vi "Sort single measurements.vi"(1 "Table In":T1[](array[typedef]) {"Carrier_2 Q (l/min)" format="%#.2f"; "Row Duration (mins)" format="%#.1f"; "Row No" min=0; "Trace Gas Concentration (%)" min=0.0 format="%#_4f"; "Carrier_1 Q (l/min)" format="%#.2f"; "Tunnel Speed" format="%#.2f"; "Start X" format="%#.2f"; "Start Y" format="%#.2f"; "Start Z" format="%#.2f"; "End X" format="%#.2f"; "End Y" format="%#.2f"; "End Z" format="%#.2f"; "Averaging time (min)" min=0.0 format="%#.2f"}) -> (0 "Table Out":T1[](array[typedef]) {"Carrier_2 Q (l/min)" format="%#.2f"; "Row Duration (mins)" format="%#.1f"; "Row No" min=0; "Trace Gas Concentration (%)" min=0.0 format="%#_4f"; "Carrier_1 Q (l/min)" format="%#.2f"; "Tunnel Speed" format="%#.2f"; "Start X" format="%#.2f"; "Start Y" format="%#.2f"; "Start Z" format="%#.2f"; "End X" format="%#.2f"; "End Y" format="%#.2f"; "End Z" format="%#.2f"; "Averaging time (min)" min=0.0 format="%#.2f"})   [LabVIEW 2014]
uses:
  Anemometry Sub Vis/Gen Trav/Traverse_cluster.ctl
  Anemometry Sub Vis/Gen Trav/Spacing.ctl
  Anemometry Sub Vis/Controls/Multi_run_mode.ctl
panel:
  out "Stop":i32[](array[numeric])
  out "Start":i32[](array[numeric])
  # "X           Y            Z"
  # "Start"
  # "End"
  # "X           Y            Z"
  # "Start"
  # "End"
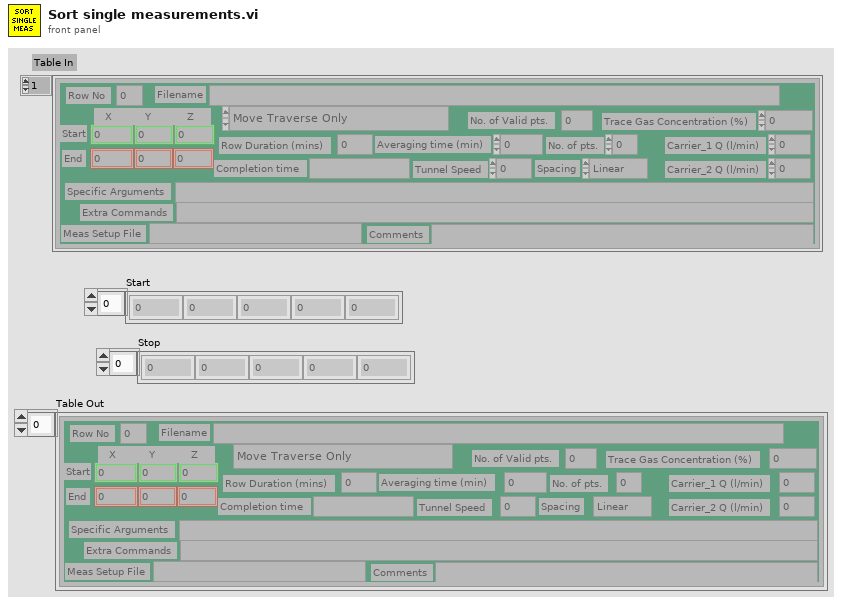
[diagram p1: front panel]
types:
  T1 = typedef "Traverse_cluster.ctl" = cluster{"Start X":sgl, "Start Y":sgl, "Start Z":sgl, "End X":sgl, "End Y":sgl, "End Z":sgl, "No. of pts.":i32, "Spacing":T2, "Filename":path, "Tunnel Speed":dbl, "Averaging time (min)":dbl, "Extra Commands":string, "Carrier_1 Q (l/min)":dbl, "Carrier_2 Q (l/min)":dbl, "Trace Gas Concentration (%)":dbl, "Specific Arguments":string, "Comments":string, "Row No":i32, "Row Type Selector":T3, "Completion time":string, "Row Duration (mins)":dbl, "No. of Valid pts.":i32, "Meas Setup File":string}
  T2 = typedef "Spacing.ctl" = enum16{"Linear", "Log", "Gauss", "Specified", "N/A"}
  T3 = typedef "Multi_run_mode.ctl" = enum16{"Move Traverse Only", "Set Tunnel Speed Only", "Set Source Only", "Set Measurement Conditions", "Single Measurement", "Vertical Profile", "Lateral Profile", "Longitudinal Profile", "Explore Volume", "Multi-Axis Profile", "Auto Calibrate", "Meas Fast FID Bkgnd", "Check Beam Power", "Scanning Valve Measurement", "Run VI Named:", "Set ADAM Ch", "Wait (minutes)", "Send Message", "Synchronize With:", "Fall Back to this Row", "Turn Off Row Repeating", "Blank Row", "Traverse 3D Volume"}
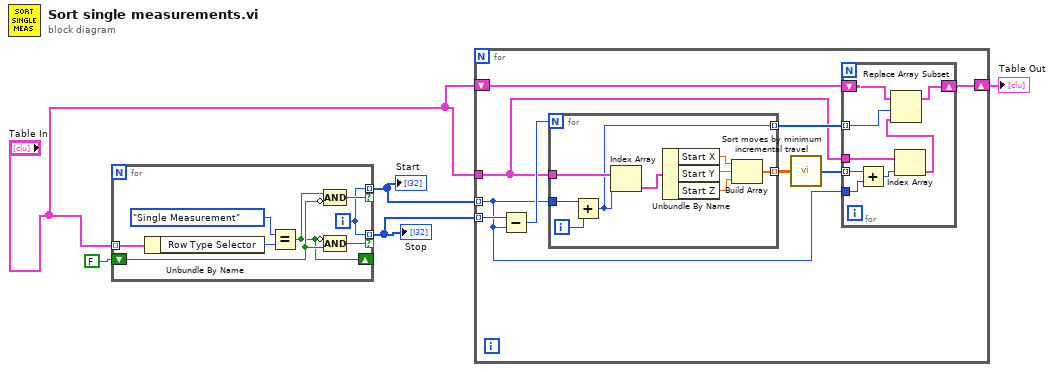
[diagram p0: block diagram]
diagram:
  n1 = for {
    tunnel: "Table In" -> [w13] mode=indexing
    shift-right: [w9] -> _
    shift-left: FALSE -> [w10]
    tunnel: [w7] -> w4 mode=indexing if=w8
    tunnel: [w7] -> w3 mode=indexing if=w6
    i -> [w7]
    n2 = Unbundle By Name(w13) -> ("Row Type Selector"=w11:T3)
    n3 = Equal?(x=Multi_run_mode."Single Measurement" ("Row Type Selector"), y=w11) -> (x = y?=w9:bool)
    n4 = Compound Arithmetic op=AND(w9, invert w10) -> (w8:bool)
    n5 = Compound Arithmetic op=AND(invert w9, w10) -> (w6:bool)
  }
  "Start" <- w4
  "Stop" <- w3
  n6 = for {
    tunnel: "Table In" -> [w15]
    tunnel: w4 -> [w14] mode=indexing
    tunnel: w3 -> [w22] mode=indexing
    shift-right: [w17] -> w1
    shift-left: "Table In" -> [w18]
    n7 = Subtract(x=w22, y=w14) -> (x-y=w21:i32)
    n8 = for {
      N: w21 -> [_]
      tunnel: w15 -> [w39]
      tunnel: w14 -> [w37]
      tunnel: [w32] -> w20 mode=indexing
      tunnel: [w31] -> w19 mode=indexing
      i -> [w38]
      n9 = Add(x=w37, y=w38) -> (x+y=w31:i32)
      n10 = Index Array(array=w39, index=w31) -> (element=w36:T1)
      n11 = Unbundle By Name(w36) -> ("Start X"=w35:sgl, "Start Y"=w34:sgl, "Start Z"=w33:sgl)
      n12 = Build Array(w35, w34, w33) -> (w32:sgl[])
    }
    n13 = call "Sort moves by minimum incremental travel.vi"("Coordinates to move through"=w20) -> ("Indices sorted by minimum incremental travel distance"=w16:i32[])
    n14 = for {
      tunnel: w19 -> [w30] mode=indexing
      shift-right: [w28] -> w17
      shift-left: w18 -> [w29]
      tunnel: w16 -> [w25] mode=indexing
      tunnel: w15 -> [w27]
      tunnel: w14 -> [w23]
      n15 = Add(x=w25, y=w23) -> (x+y=w24:i32)
      n16 = Index Array(array=w27, index=w24) -> (element=w26:T1)
      n17 = Replace Array Subset(array=w29, new element=w26, index=w30) -> (w28:T1[])
    }
  }
  "Table Out" <- w1
